vi "Enter_LDA_Setup.vi"(0 "Show Panel":bool) -> ()   [LabVIEW 2010]
uses:
  Controls/BSA_info_Cluster.ctl
  BSA_Type.ctl
  Globals/Constants_global.vi
  Globals/LDA_meas_global_1.vi
  Globals/LDA_meas_global_2.vi
panel:
  in  "Blue Shifted":i32
  in  "Blue Unshifted":i32
  in  "Green Shifted":i32
  in  "Green Unshifted":i32
  in  "BSA Type":T1
  in  "BSA IP Number":string
  in  "Beam Alignment":u16(ring) items=["No Info", "Tunnel", "Model"]
  in  "45 Degree Mirror":bool
  in  "Swap BSA Order":bool
  in  "BSA Info":T2[](array[typedef]) {"Wavelength (nm)" format="%.1f"}
  in  "Probe Type":u16(ring) items=["14mm probe; Beam Separation=8mm; Focal Length=50mm", "14mm probe with beam expander; Beam Separation=16mm; Focal Length=120mm", "Test; Beam Separation=14mm; Focal Length=20mm", "Add Another LDA Probe"]
  in  "OK":bool
  # "Warn if Power below (mW)"
  # "BSA 1"
  # "BSA 2"
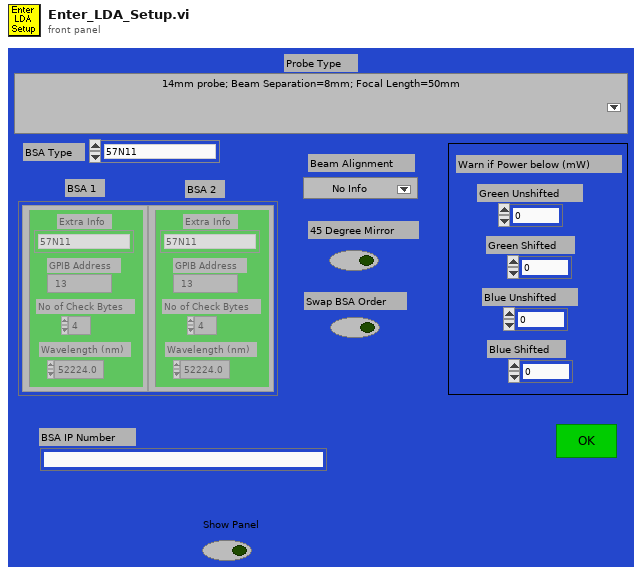
[diagram p1: front panel]
types:
  T1 = typedef "BSA_Type.ctl" = enum16{"57N11", "BSA F60"}
  T2 = typedef "BSA_info_Cluster.ctl" = cluster{"GPIB Address":string, "No of Check Bytes":i32, "Extra Info":string, "COLOUR":u32, "Wavelength (nm)":dbl}
  T3 = cluster{"Probe Name":string, "Beam Separation (mm)":dbl, "Focal Length (mm)":dbl}
  T4 = cluster{"Probe Name":string, "Beam Separation (mm)":dbl, "Focal Length (mm)":dbl}[]
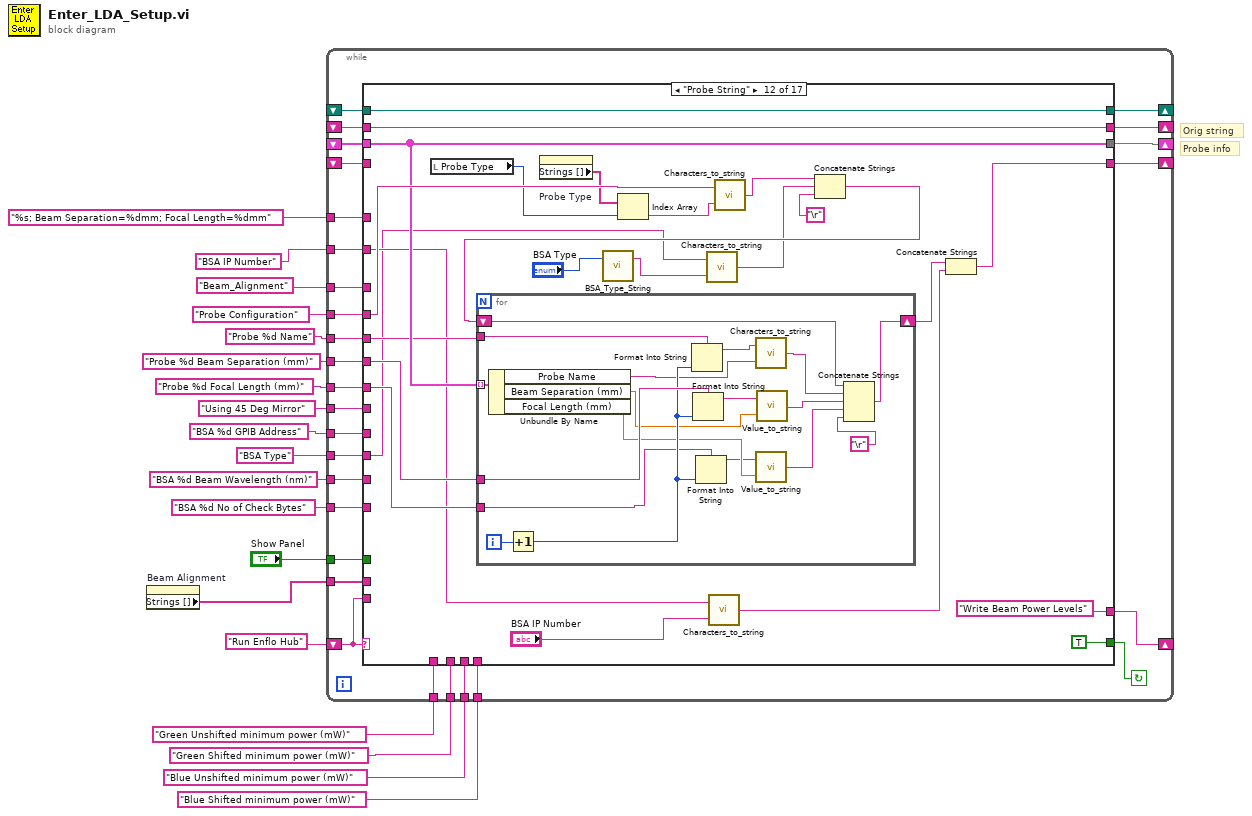
[diagram p0: block diagram]
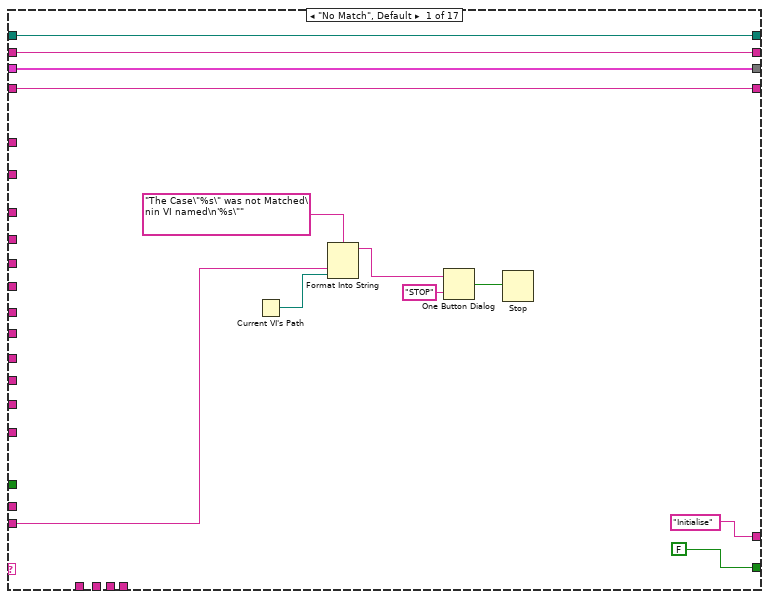
[diagram p2: hidden frame]
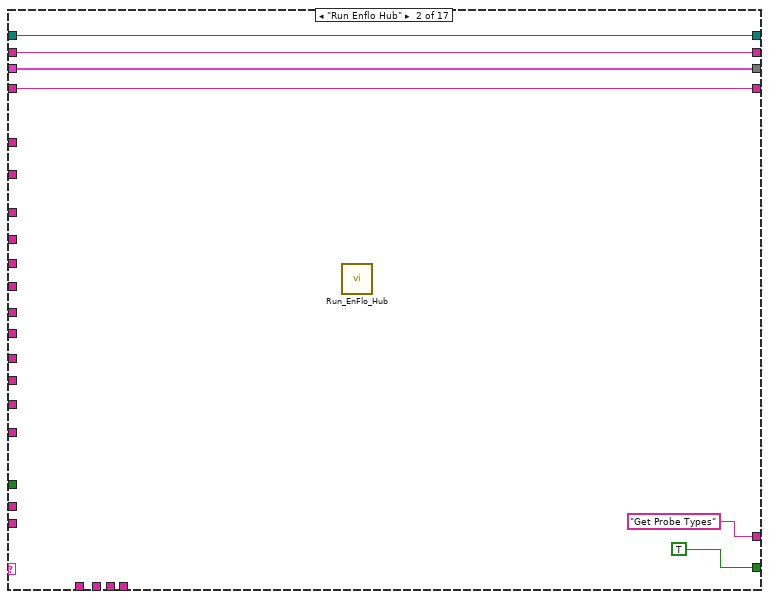
[diagram p3: hidden frame]
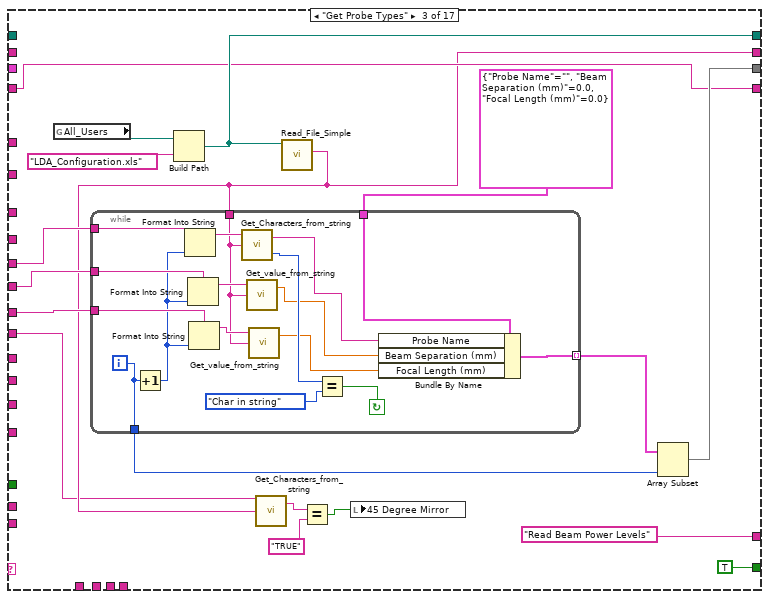
[diagram p4: hidden frame]
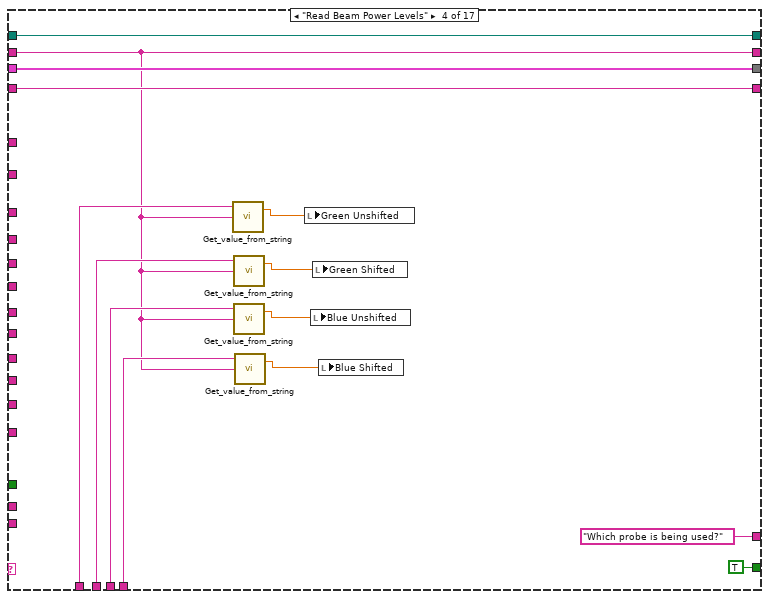
[diagram p5: hidden frame]
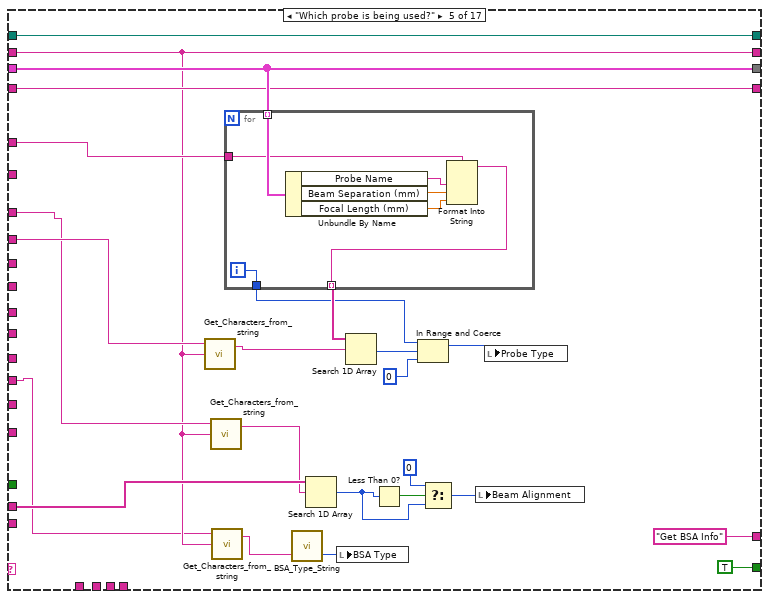
[diagram p6: hidden frame]
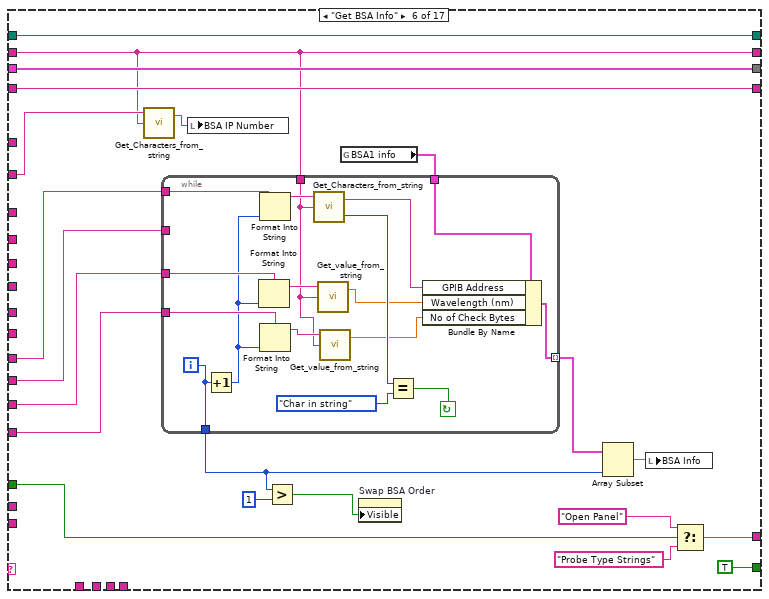
[diagram p7: hidden frame]
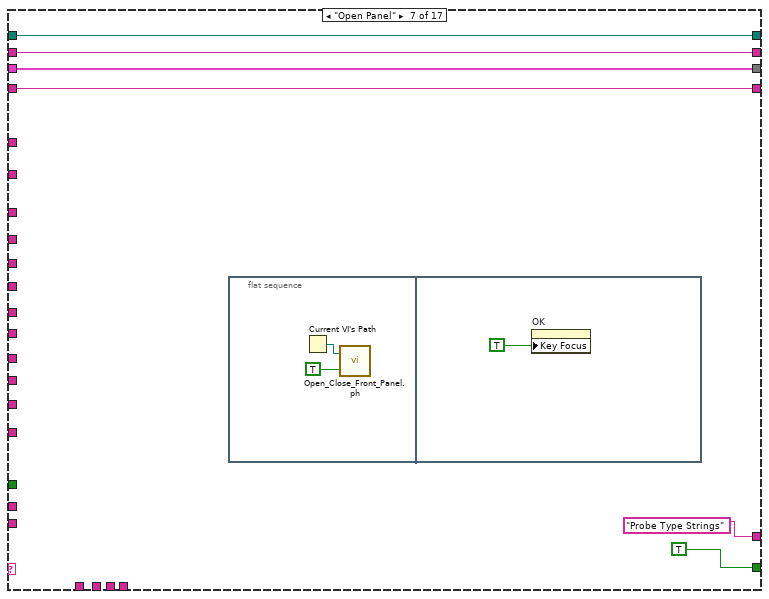
[diagram p8: hidden frame]
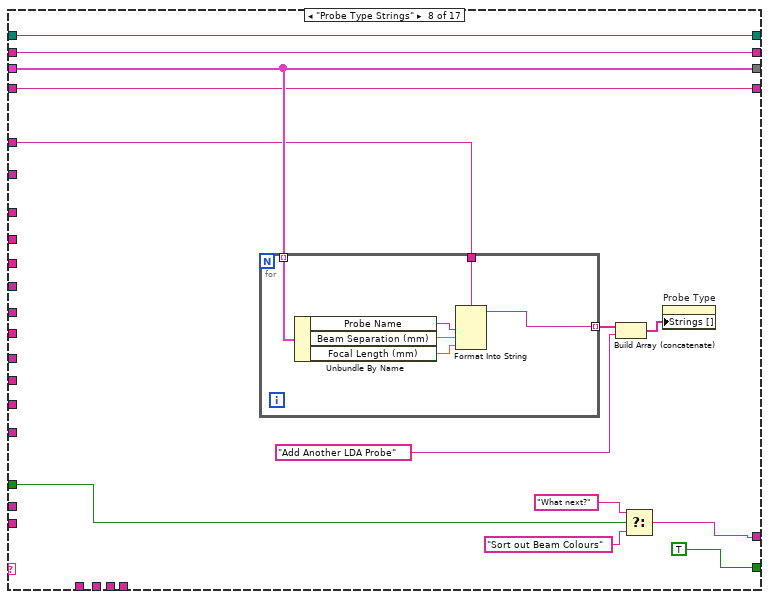
[diagram p9: hidden frame]
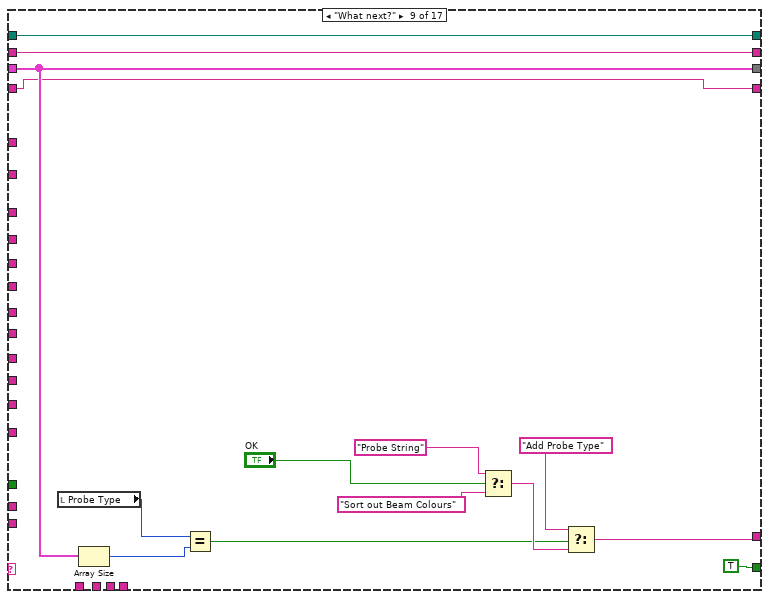
[diagram p10: hidden frame]
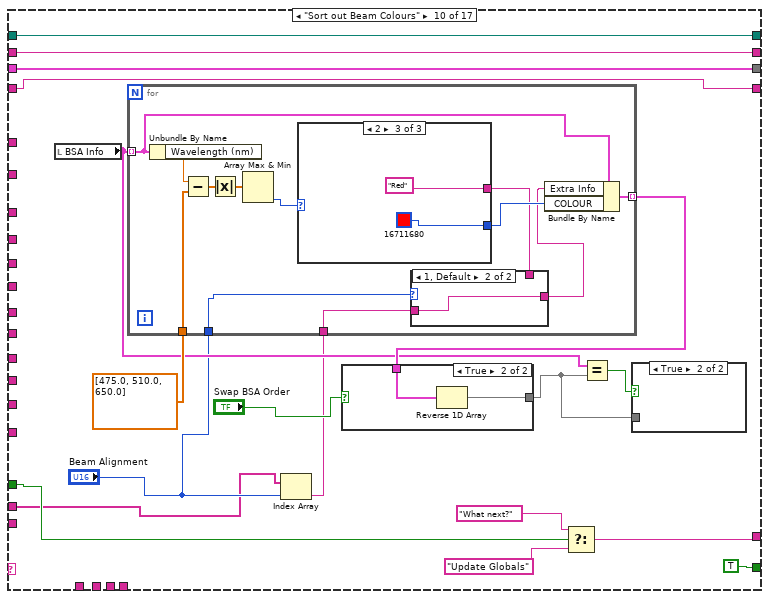
[diagram p11: hidden frame]
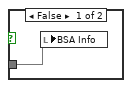
[diagram p12: hidden frame]
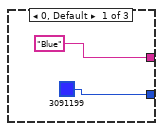
[diagram p15: hidden frame]
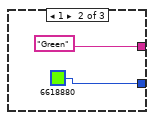
[diagram p16: hidden frame]
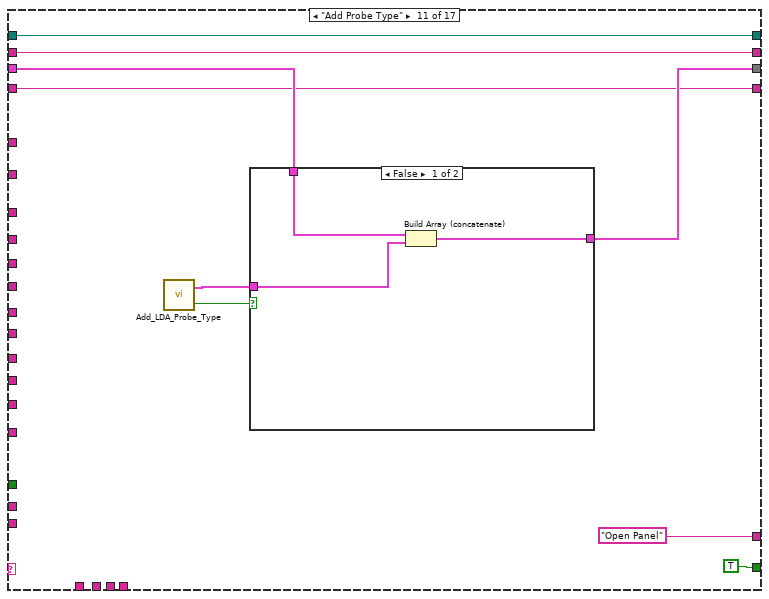
[diagram p17: hidden frame]
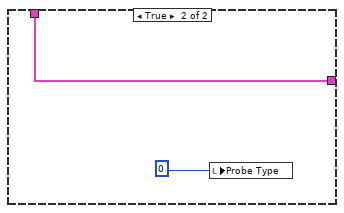
[diagram p18: hidden frame]
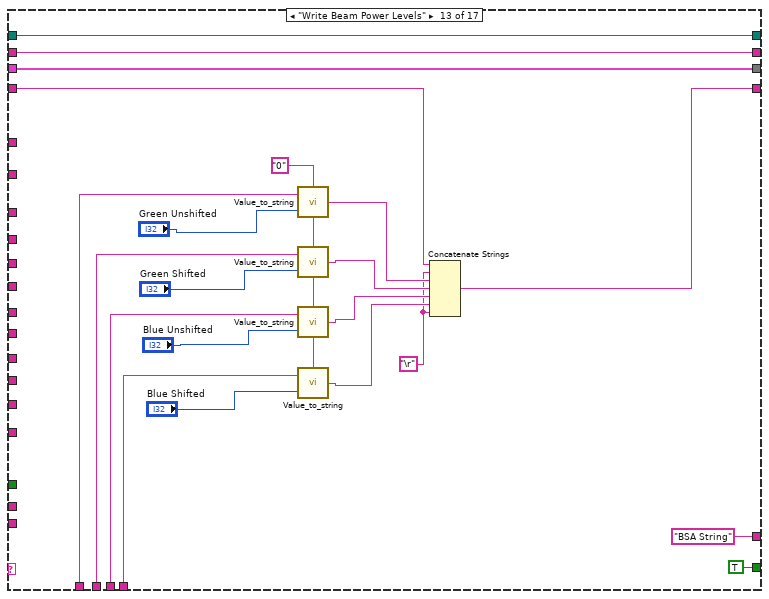
[diagram p19: hidden frame]
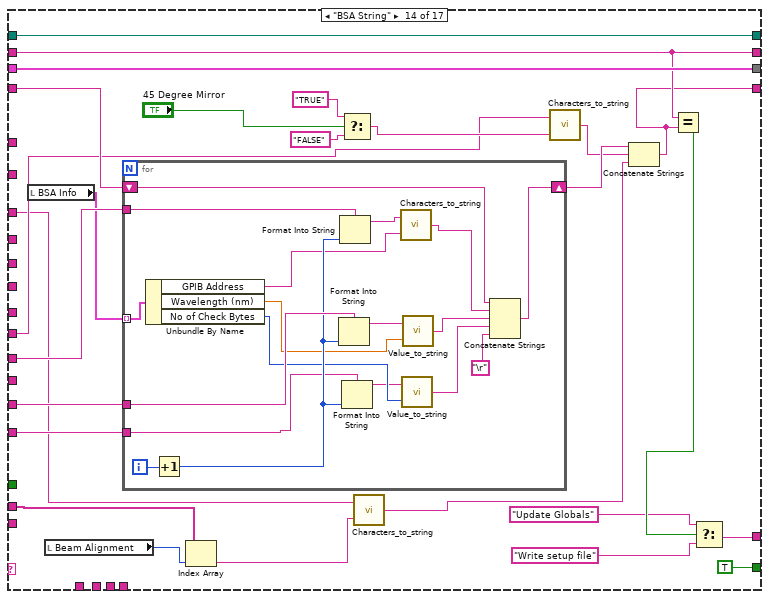
[diagram p20: hidden frame]
diagram:
  # "Orig string"
  # "Probe info"
  n1 = property on="Beam Alignment" class="Ring (strict)"() -> ("Strings []"=w7:string[])  [unwired: 2 in, 2 out]
  n2 = while {
    shift-left: "Run Enflo Hub" -> [w46]
    shift-right: [w47] -> _
    shift-right: [w45] -> _
    shift-left: _ -> [w44]
    tunnel: "Probe %d Name" -> [w43]
    shift-right: [w42] -> _
    shift-left: _ -> [w38]
    tunnel: "Probe %d Focal Length (mm)" -> [w41]
    tunnel: "Probe %d Beam Separation (mm)" -> [w40]
    shift-right: [w39] -> _
    shift-left: _ -> [w37]
    tunnel: "Probe Configuration" -> [w36]
    tunnel: "Show Panel" -> [w35]
    tunnel: "BSA %d GPIB Address" -> [w34]
    tunnel: "BSA Type" -> [w33]
    tunnel: "BSA %d Beam Wavelength (nm)" -> [w32]
    tunnel: "BSA %d No of Check Bytes" -> [w31]
    shift-right: [w29] -> _
    shift-left: _ -> [w30]
    tunnel: "%s; Beam Separation=%dmm; Focal Length=%dmm" ("format string") -> [w28]
    tunnel: "Using 45 Deg Mirror" -> [w27]
    tunnel: w7 -> [w26]
    tunnel: "Beam_Alignment" -> [w25]
    tunnel: "BSA IP Number" -> [w24]
    tunnel: "Green Unshifted minimum power (mW)" -> [w23]
    tunnel: "Green Shifted minimum power (mW)" -> [w22]
    tunnel: "Blue Unshifted minimum power (mW)" -> [w21]
    tunnel: "Blue Shifted minimum power (mW)" -> [w20]
    stop <- w48 continue-if-true
    n3 = case shown="\"Probe String\"" w46 {
      tunnel: [FALSE TRUE TRUE TRUE ("Show Panel") TRUE TRUE TRUE TRUE TRUE TRUE TRUE TRUE TRUE ("Show Panel") TRUE TRUE w414 FALSE] -> w48
      tunnel: ["Initialise" "Get Probe Types" "Read Beam Power Levels" "Which probe is being used?" "Get BSA Info" w163 "Probe Type Strings" w195 w220 w239 "Open Panel" ("f") "Write Beam Power Levels" "BSA String" w359 "Update Globals" "Close Panel" "End"] -> w47
      tunnel: w46 -> [w55 _ _ _ _ _ _ _ _ _ _ _ _ _ _ _ _]
      tunnel: [w52 w64 w80 w113 w136 w157 w188 w205 w224 w243 w276 w305 w343 w367 w395 w422 w428] -> w45
      tunnel: w44 -> [w52 w64 _ w113 w136 w157 w188 w205 w224 w243 w276 w305 w343 w367 w395 w422 w428]
      tunnel: w43 -> [_ _ w81 _ _ _ _ _ _ _ _ w298 _ _ _ _ _]
      tunnel: [w51 w63 w71 w102 w119 w148 w187 w204 w222 w242 w275 w300 w341 w363 w394 w421 w425] -> w42
      tunnel: w41 -> [_ _ w79 _ _ _ _ _ _ _ _ w296 _ _ _ _ _]
      tunnel: w40 -> [_ _ w78 _ _ _ _ _ _ _ _ w297 _ _ _ _ _]
      tunnel: [w50 w62 w74 w112 w135 w156 w186 w203 w218 w238 w270 w299 w342 w366 w396 w417 w424] -> w39
      tunnel: w38 -> [w51 w63 _ w102 w119 w148 w187 w204 w222 w242 w275 w300 w341 w363 w394 w421 w425]
      tunnel: w37 -> [w50 w62 _ w112 w135 w156 w186 w203 w218 w238 w271 w299 w342 w366 w396 w417 w424]
      tunnel: w36 -> [_ _ _ _ w137 _ _ _ _ _ _ w304 _ _ _ _ _]
      tunnel: w35 -> [_ _ _ _ _ w165 _ w196 _ w232 _ _ _ _ _ w414 _]
      tunnel: w34 -> [_ _ _ _ _ w161 _ _ _ _ _ _ _ w370 _ _ _]
      tunnel: w33 -> [_ _ _ _ w118 w160 _ _ _ _ _ w284 _ _ _ _ _]
      tunnel: w32 -> [_ _ _ _ _ w159 _ _ _ _ _ _ _ w369 _ _ _]
      tunnel: w31 -> [_ _ _ _ _ w158 _ _ _ _ _ _ _ w368 _ _ _]
      tunnel: w30 -> [w49 w61 w72 w111 w128 w150 w185 w202 w214 w237 w269 _ w326 w364 w390 w410 w423]
      tunnel: [w49 w61 w72 w111 w128 w150 w185 w202 w214 w237 w269 w289 w325 w353 w390 w410 w423] -> w29
      tunnel: w28 -> [_ _ _ _ w127 _ _ w194 _ _ _ _ _ _ _ _ _]
      tunnel: w27 -> [_ _ w67 _ _ _ _ _ _ _ _ _ _ w351 _ _ _]
      tunnel: w26 -> [_ _ _ _ w125 _ _ _ _ w227 _ _ _ w348 _ _ _]
      tunnel: w25 -> [_ _ _ _ w126 _ _ _ _ _ _ _ _ w350 _ _ _]
      tunnel: w24 -> [_ _ _ _ _ w149 _ _ _ _ _ w291 _ _ _ _ _]
      tunnel: w23 -> [_ _ _ w110 _ _ _ _ _ _ _ _ w340 _ _ _ _]
      tunnel: w22 -> [_ _ _ w105 _ _ _ _ _ _ _ _ w339 _ _ _ _]
      tunnel: w21 -> [_ _ _ w104 _ _ _ _ _ _ _ _ w338 _ _ _ _]
      tunnel: w20 -> [_ _ _ w103 _ _ _ _ _ _ _ _ w337 _ _ _ _]
      frame "No Match", Default {
        n4 = Current VI's Path() -> (path=w54:path)
        n5 = Format Into String(format string="The Case\"%s\" was not Matched\nin VI named\n'%s\"" ("Format String"), w55, w54) -> (resulting string=w58:string)  [unwired: 2 in, 1 out]
        n6 = One Button Dialog(message=w58, button name ("OK")="STOP") -> (true=w56:bool)
        n7 = Stop(stop? (T)=w56) -> ()
      }
      frame "Run Enflo Hub" {
        n8 = call "Run_EnFlo_Hub.vi"() -> ()  [unwired: 8 out]
      }
      frame "Get Probe Types" {
        n9 = global read "Constants_global.vi" "All_Users"() -> (w83:path)
        n10 = Build Path(base path=w83, name or relative path="LDA_Configuration.xls") -> (appended path=w80:path)
        n11 = call "Read_File_Simple.vi"("Filename"=w80) -> ("string"=w71:string)  [unwired: 2 in, 7 out]
        n12 = while {
          tunnel: w81 -> [w101]
          tunnel: w71 -> [w95]
          tunnel: w79 -> [w99]
          tunnel: w78 -> [w98]
          tunnel: [w90] -> w77
          tunnel: T3 {"Probe Name"="", "Beam Separation (mm)"=0.0, "Focal Length (mm)"=0.0} -> [w89]
          tunnel: [w86] -> w75 mode=indexing
          i -> [w90]
          stop <- w91 continue-if-true
          n13 = Increment(x=w90) -> (x+1=w94:i32)
          n14 = Format Into String(format string=w101, w94) -> (resulting string=w100:string)  [unwired: 2 in, 1 out]
          n15 = Format Into String(format string=w98, w94) -> (resulting string=w97:string)  [unwired: 2 in, 1 out]
          n16 = Format Into String(format string=w99, w94) -> (resulting string=w96:string)  [unwired: 2 in, 1 out]
          n17 = call "Get_Characters_from_string.vi"("Input string"=w95, "Variable name"=w100) -> ("Status"=w92:enum16{"Char in string", "Char not in string"}, "Value"=w85:string)  [unwired: 1 in]
          n18 = call "Get_value_from_string.vi"("Input string"=w95, "Variable name"=w97) -> ("Value"=w87:dbl)  [unwired: 1 in, 1 out]
          n19 = call "Get_value_from_string.vi"("Input string"=w95, "Variable name"=w96) -> ("Value"=w88:dbl)  [unwired: 1 in, 1 out]
          n20 = Equal?(x=w92, y=enum16{"Char in string", "Char not in string"}."Char in string" ("Status")) -> (x = y?=w91:bool)
          n21 = Bundle By Name(cluster=w89, "Probe Name"=w85, "Beam Separation (mm)"=w87, "Focal Length (mm)"=w88) -> (w86:T3)
        }
        n22 = call "Get_Characters_from_string.vi"("Input string"=w71, "Variable name"=w67) -> ("Value"=w70:string)  [unwired: 1 in, 1 out]
        n23 = Equal?(x=w70, y="TRUE") -> (x = y?=w68:bool)
        n24 = local write "45 Degree Mirror"(w68) -> ()
        n25 = Array Subset(array=w75, length=w77) -> (w74:T4)  [unwired: 1 in]
      }
      frame "Read Beam Power Levels" {
        n26 = call "Get_value_from_string.vi"("Input string"=w102, "Variable name"=w110) -> ("Value"=w109:dbl)  [unwired: 1 in, 1 out]
        n27 = call "Get_value_from_string.vi"("Input string"=w102, "Variable name"=w105) -> ("Value"=w108:dbl)  [unwired: 1 in, 1 out]
        n28 = call "Get_value_from_string.vi"("Input string"=w102, "Variable name"=w104) -> ("Value"=w107:dbl)  [unwired: 1 in, 1 out]
        n29 = call "Get_value_from_string.vi"("Input string"=w102, "Variable name"=w103) -> ("Value"=w106:dbl)  [unwired: 1 in, 1 out]
        n30 = local write "Green Unshifted"(w109) -> ()
        n31 = local write "Blue Unshifted"(w107) -> ()
        n32 = local write "Green Shifted"(w108) -> ()
        n33 = local write "Blue Shifted"(w106) -> ()
      }
      frame "Which probe is being used?" {
        n34 = call "Get_Characters_from_string.vi"("Input string"=w119, "Variable name"=w137) -> ("Value"=w133:string)  [unwired: 1 in, 1 out]
        n35 = call "Get_Characters_from_string.vi"("Input string"=w119, "Variable name"=w126) -> ("Value"=w124:string)  [unwired: 1 in, 1 out]
        n36 = call "Get_Characters_from_string.vi"("Input string"=w119, "Variable name"=w118) -> ("Value"=w117:string)  [unwired: 1 in, 1 out]
        n37 = for {
          tunnel: w135 -> [w142] mode=indexing
          tunnel: [w140] -> w134 mode=indexing
          tunnel: [w146] -> w131
          tunnel: w127 -> [w141]
          i -> [w146]
          n38 = Unbundle By Name(w142) -> ("Probe Name"=w143:string, "Beam Separation (mm)"=w144:dbl, "Focal Length (mm)"=w145:dbl)
          n39 = Format Into String(format string=w141, w143, w144, w145) -> (resulting string=w140:string)  [unwired: 2 in, 1 out]
        }
        n40 = call "BSA_Type_String.vi"("BSA String in"=w117) -> ("BSA Type Out"=w116:T1)  [unwired: 1 in, 1 out]
        n41 = Search 1D Array(1D array=w125, element=w124) -> (index of element=w121:i32)  [unwired: 1 out]
        n42 = local write "BSA Type"(w116) -> ()
        n43 = Search 1D Array(1D array=w134, element=w133) -> (index of element=w132:i32)  [unwired: 1 out]
        n44 = Less Than 0?(x=w121) -> (x < 0?=w123:bool)
        n45 = In Range and Coerce(upper limit=w131, x=w132, lower limit=0) -> (coerced(x)=w129:i32)  [unwired: 1 out]
        n46 = Select(t=0, s=w123, f=w121) -> (s? t:f=w120:i32)
        n47 = local write "Beam Alignment"(w120) -> ()
        n48 = local write "Probe Type"(w129) -> ()
      }
      frame "Get BSA Info" {
        n49 = call "Get_Characters_from_string.vi"("Input string"=w148, "Variable name"=w149) -> ("Value"=w147:string)  [unwired: 1 in, 1 out]
        n50 = local write "BSA IP Number"(w147) -> ()
        n51 = global read "LDA_meas_global_1.vi" "BSA1 info"() -> (w162:T2)
        n52 = while {
          tunnel: w160 -> [_]
          tunnel: w148 -> [w168]
          tunnel: w158 -> [w184]
          tunnel: w159 -> [w183]
          tunnel: [w178] -> w153
          tunnel: w162 -> [w177]
          tunnel: [w176] -> w166 mode=indexing
          tunnel: w161 -> [w173]
          i -> [w178]
          stop <- w179 continue-if-true
          n53 = Increment(x=w178) -> (x+1=w174:i32)
          n54 = Format Into String(format string=w183, w174) -> (resulting string=w182:string)  [unwired: 2 in, 1 out]
          n55 = Format Into String(format string=w173, w174) -> (resulting string=w175:string)  [unwired: 2 in, 1 out]
          n56 = Format Into String(format string=w184, w174) -> (resulting string=w181:string)  [unwired: 2 in, 1 out]
          n57 = call "Get_Characters_from_string.vi"("Input string"=w168, "Variable name"=w175) -> ("Status"=w172:enum16{"Char in string", "Char not in string"}, "Value"=w171:string)  [unwired: 1 in]
          n58 = call "Get_value_from_string.vi"("Input string"=w168, "Variable name"=w182) -> ("Value"=w170:dbl)  [unwired: 1 in, 1 out]
          n59 = call "Get_value_from_string.vi"("Input string"=w168, "Variable name"=w181) -> ("Value"=w169:dbl)  [unwired: 1 in, 1 out]
          n60 = Equal?(x=w172, y=enum16{"Char in string", "Char not in string"}."Char in string" ("Status")) -> (x = y?=w179:bool)
          n61 = Bundle By Name(cluster=w177, "GPIB Address"=w171, "Wavelength (nm)"=w170, "No of Check Bytes"=w169) -> (w176:T2)
        }
        n62 = Greater?(x=w153, y=1) -> (0:w151:bool)
        n63 = property on="Swap BSA Order" class="Bool"("Visible"=w151) -> ()  [unwired: 2 in, 2 out]
        n64 = Array Subset(array=w166, length=w153) -> (w155:T2[])  [unwired: 1 in]
        n65 = local write "BSA Info"(w155) -> ()
        n66 = Select(t="Open Panel", s=w165, f="Probe Type Strings") -> (s? t:f=w163:string)
      }
      frame "Open Panel" {
        n67 = flat-sequence {
          frame #0 {
            n68 = Current VI's Path() -> (path=w192:path)
            n69 = call "Open_Close_Front_Panel.ph.vi"("Front Panel Window:Open"=TRUE, "VI path"=w192) -> ()  [unwired: 2 out]
          }
          frame #1 {
            n70 = property on="OK" class="Bool"("Key Focus"=TRUE) -> ()  [unwired: 2 in, 2 out]
          }
        }
      }
      frame "Probe Type Strings" {
        n71 = for {
          tunnel: w203 -> [w212] mode=indexing
          tunnel: [w211] -> w201 mode=indexing
          tunnel: w194 -> [w207]
          n72 = Unbundle By Name(w212) -> ("Probe Name"=w210:string, "Beam Separation (mm)"=w209:dbl, "Focal Length (mm)"=w208:dbl)
          n73 = Format Into String(format string=w207, w210, w209, w208) -> (resulting string=w211:string)  [unwired: 2 in, 1 out]
        }
        n74 = Build Array (concatenate)(w201, "Add Another LDA Probe" ("Probe Name")) -> (w200:string[])
        n75 = Select(t="What next?", s=w196, f="Sort out Beam Colours") -> (s? t:f=w195:string)
        n76 = property on="Probe Type" class="Ring (strict)"("Strings []"=w200) -> ()  [unwired: 2 in, 2 out]
      }
      frame "What next?" {
        n77 = local read "Probe Type"() -> (w216:u16)
        n78 = Array Size(array=w218) -> (size(s)=w217:i32)
        n79 = Equal?(x=w216, y=w217) -> (x = y?=w215:bool)
        n80 = Select(t="Probe String", s="OK", f="Sort out Beam Colours") -> (s? t:f=w221:string)
        n81 = Select(t="Add Probe Type", s=w215, f=w221) -> (s? t:f=w220:string)
      }
      frame "Sort out Beam Colours" {
        n82 = local read "BSA Info"() -> (w236:T2[])
        n83 = Index Array(array=w227, index="Beam Alignment") -> (element=w228:string)
        n84 = for {
          tunnel: w236 -> [w255] mode=indexing
          tunnel: dbl[] [475.0, 510.0, 650.0] -> [w259]
          tunnel: [w253] -> w240 mode=indexing
          tunnel: "Beam Alignment" -> [w252]
          tunnel: w228 -> [w249]
          n85 = Unbundle By Name(w255) -> ("Wavelength (nm)"=w260:dbl)
          n86 = Subtract(x=w260, y=w259) -> (x-y=w258:dbl[])
          n87 = Absolute Value(x=w258) -> (abs(x)=w257:dbl[])
          n88 = Array Max & Min(array=w257) -> (min index (indices)=w256:i32)  [unwired: 3 out]
          n89 = case shown="2" w256 {
            tunnel: ["Blue" "Green" "Red"] -> w250
            tunnel: [u32 3091199 u32 6618880 u32 16711680] -> w254
            frame 0, Default {
            }
            frame 1 {
            }
            frame 2 {
            }
          }
          n90 = case shown="1, Default" w252 {
            tunnel: [w261 w262] -> w251
            tunnel: w250 -> [w261 _]
            tunnel: w249 -> [_ w262]
            frame 0 {
            }
            frame 1, Default {
            }
          }
          n91 = Bundle By Name(cluster=w255, "Extra Info"=w251, "COLOUR"=w254) -> (w253:T2)
        }
        n92 = case shown="True" "Swap BSA Order" {
          tunnel: w240 -> [w246 w248]
          tunnel: [w246 w247] -> w234
          frame False {
          }
          frame True {
            n93 = Reverse 1D Array(array=w248) -> (reversed array=w247:T2[])
          }
        }
        n94 = Select(t="What next?" ("f"), s=w232, f="Update Globals") -> (s? t:f=w239:string)
        n95 = Equal?(x=w236, y=w234) -> (x = y?=w235:bool)
        n96 = case shown="True" w235 {
          tunnel: w234 -> [w245 _]
          frame False {
            n97 = local write "BSA Info"(w245) -> ()
          }
          frame True {
          }
        }
      }
      frame "Add Probe Type" {
        n98 = call "Add_LDA_Probe_Type.vi"() -> ("Cancel Out"=w273:bool, "New LDA Probe Type Out"=w272:T3)  [unwired: 3 out]
        n99 = case shown="False" w273 {
          tunnel: w272 -> [w280 _]
          tunnel: w271 -> [w279 w282]
          tunnel: [w278 w282] -> w270
          frame False {
            n100 = Build Array (concatenate)(w279, w280) -> (w278:T4)
          }
          frame True {
            n101 = local write "Probe Type"(0) -> ()
          }
        }
      }
      frame "Probe String" {
        n102 = local read "Probe Type"() -> (w293:u16)
        n103 = property on="Probe Type" class="Ring (strict)"() -> ("Strings []"=w294:string[])  [unwired: 2 in, 2 out]
        n104 = call "BSA_Type_String.vi"("BSA Type"="BSA Type") -> ("BSA String Out"=w285:string)  [unwired: 1 in, 1 out]
        n105 = Index Array(array=w294, index=w293) -> (element=w292:string)
        n106 = call "Characters_to_string.vi"("Characters to write"=w285, "Label for characters"=w284) -> ("Output string"=w283:string)
        n107 = call "Characters_to_string.vi"("Characters to write"="BSA IP Number", "Label for characters"=w291) -> ("Output string"=w288:string)
        n108 = call "Characters_to_string.vi"("Characters to write"=w292, "Label for characters"=w304) -> ("Output string"=w303:string)
        n109 = Concatenate Strings(w303, w283, "\r") -> (w301:string)
        n110 = for {
          tunnel: w298 -> [w323]
          tunnel: w297 -> [w322]
          tunnel: w296 -> [w320]
          shift-right: [w316] -> w290
          shift-left: w301 -> [w308]
          tunnel: w299 -> [w309] mode=indexing
          i -> [w324]
          n111 = Unbundle By Name(w309) -> ("Probe Name"=w315:string, "Beam Separation (mm)"=w314:dbl, "Focal Length (mm)"=w313:dbl)
          n112 = Increment(x=w324) -> (x+1=w321:i32)
          n113 = Format Into String(format string=w323, w321) -> (resulting string=w310:string)  [unwired: 2 in, 1 out]
          n114 = Format Into String(format string=w322, w321) -> (resulting string=w311:string)  [unwired: 2 in, 1 out]
          n115 = Format Into String(format string=w320, w321) -> (resulting string=w312:string)  [unwired: 2 in, 1 out]
          n116 = call "Characters_to_string.vi"("Characters to write"=w315, "Label for characters"=w310) -> ("Output string"=w317:string)
          n117 = call "Value_to_string.vi"("Value"=w313, "Label for value"=w312) -> ("Output string"=w319:string)  [unwired: 1 in]
          n118 = call "Value_to_string.vi"("Value"=w314, "Label for value"=w311) -> ("Output string"=w318:string)  [unwired: 1 in]
          n119 = Concatenate Strings(w308, w317, w318, w319, "\r") -> (w316:string)
        }
        n120 = Concatenate Strings(w290, w288) -> (w289:string)
      }
      frame "Write Beam Power Levels" {
        w327 = "\r"
        w336 = "0" ("precision")
        n121 = call "Value_to_string.vi"("precision"=w336, "Value"="Green Unshifted", "Label for value"=w340) -> ("Output string"=w331:string)
        n122 = call "Value_to_string.vi"("precision"=w336, "Value"="Green Shifted", "Label for value"=w339) -> ("Output string"=w330:string)
        n123 = call "Value_to_string.vi"("precision"=w336, "Value"="Blue Unshifted", "Label for value"=w338) -> ("Output string"=w329:string)
        n124 = call "Value_to_string.vi"("precision"=w336, "Value"="Blue Shifted", "Label for value"=w337) -> ("Output string"=w328:string)
        n125 = Concatenate Strings(w326, w327, w331, w330, w329, w328, w327) -> (w325:string)
      }
      frame "BSA String" {
        n126 = local read "BSA Info"() -> (w365:T2[])
        n127 = local read "Beam Alignment"() -> (w349:u16)
        n128 = for {
          tunnel: w370 -> [w388]
          tunnel: w369 -> [w387]
          tunnel: w368 -> [w385]
          shift-right: [w380] -> w354
          shift-left: w364 -> [w373]
          tunnel: w365 -> [w384] mode=indexing
          i -> [w389]
          n129 = Unbundle By Name(w384) -> ("GPIB Address"=w378:string, "Wavelength (nm)"=w377:dbl, "No of Check Bytes"=w376:i32)
          n130 = Increment(x=w389) -> (x+1=w386:i32)
          n131 = Format Into String(format string=w387, w386) -> (resulting string=w374:string)  [unwired: 2 in, 1 out]
          n132 = Format Into String(format string=w388, w386) -> (resulting string=w379:string)  [unwired: 2 in, 1 out]
          n133 = Format Into String(format string=w385, w386) -> (resulting string=w375:string)  [unwired: 2 in, 1 out]
          n134 = call "Characters_to_string.vi"("Characters to write"=w378, "Label for characters"=w379) -> ("Output string"=w381:string)
          n135 = call "Value_to_string.vi"("Value"=w376, "Label for value"=w375) -> ("Output string"=w383:string)  [unwired: 1 in]
          n136 = call "Value_to_string.vi"("Value"=w377, "Label for value"=w374) -> ("Output string"=w382:string)  [unwired: 1 in]
          n137 = Concatenate Strings(w373, w381, w382, w383, "\r") -> (w380:string)
        }
        n138 = Index Array(array=w348, index=w349) -> (element=w347:string)
        n139 = Select(t="TRUE", s="45 Degree Mirror", f="FALSE") -> (s? t:f=w355:string)
        n140 = call "Characters_to_string.vi"("Characters to write"=w347, "Label for characters"=w350) -> ("Output string"=w346:string)
        n141 = call "Characters_to_string.vi"("Characters to write"=w355, "Label for characters"=w351) -> ("Output string"=w352:string)
        n142 = Concatenate Strings(w354, w352, w346) -> (w353:string)
        n143 = Equal?(x=w363, y=w353) -> (x = y?=w362:bool)
        n144 = Select(t="Update Globals", s=w362, f="Write setup file") -> (s? t:f=w359:string)
      }
      frame "Write setup file" {
        w392 = FALSE  # append to file? (new file:F)
        w393 = FALSE  # advisory dialog? (display:T)
        n145 = call "Write_Characters_To_File.vi"("file path (dialog if empty)"=w395, "advisory dialog? (display:T)"=w393, "character string"=w390, "append to file? (new file:F)"=w392) -> ()  [unwired: 1 in, 4 out]
      }
      frame "Update Globals" {
        n146 = local read "BSA Type"() -> (w402:T1)
        n147 = local read "45 Degree Mirror"() -> (w404:bool)
        n148 = Index Array(array="BSA Info", index=0) -> (element=w412:T2)
        n149 = Index Array(array="BSA Info", index=1) -> (element=w411:T2)
        n150 = Index Array(array=w417, index="Probe Type") -> (element=w418:T3)
        n151 = global write "LDA_meas_global_1.vi" "BSA Type"(w402) -> ()
        n152 = global write "LDA_meas_global_1.vi" "Using 45 Degree Mirror?"(w404) -> ()
        n153 = global write "LDA_meas_global_2.vi" "BSA2 info"(w411) -> ()
        n154 = Unbundle By Name(w418) -> ("Probe Name"=w406:string, "Beam Separation (mm)"=w407:dbl, "Focal Length (mm)"=w408:dbl)
        n155 = global write "LDA_meas_global_1.vi" "BSA1 info"(w412) -> ()
        n156 = local read "BSA IP Number"() -> (w403:string)
        n157 = local read "Green Unshifted"() -> (w401:i32)
        n158 = local read "Blue Unshifted"() -> (w399:i32)
        n159 = local read "Green Shifted"() -> (w400:i32)
        n160 = local read "Blue Shifted"() -> (w398:i32)
        n161 = global write "LDA_meas_global_1.vi" "Beam Separation (mm)"(w407) -> ()
        n162 = global write "LDA_meas_global_1.vi" "BSA IP Number"(w403) -> ()
        n163 = global write "LDA_meas_global_1.vi" "Focal Length (mm)"(w408) -> ()
        n164 = Format Into String(format string="%s; Beam Separation=%dmm; Focal Length=%dmm", w406, w407, w408) -> (resulting string=w405:string)  [unwired: 2 in, 1 out]
        n165 = global write "LDA_meas_global_1.vi" "Min Green Unshifted Power mW"(w401) -> ()
        n166 = global write "LDA_meas_global_1.vi" "Min Blue Unshifted Power mW"(w399) -> ()
        n167 = global write "LDA_meas_global_1.vi" "Min Green Shifted Power mW"(w400) -> ()
        n168 = global write "LDA_meas_global_1.vi" "Min Blue Shifted Power mW"(w398) -> ()
        n169 = global write "LDA_meas_global_1.vi" "Probe Configuration"(w405) -> ()
      }
      frame "Close Panel" {
        n170 = Current VI's Path() -> (path=w427:path)
        n171 = call "Open_Close_Front_Panel.ph.vi"("Front Panel Window:Open"=FALSE, "VI path"=w427) -> ()  [unwired: 2 out]
      }
    }
  }
